vi "old - RT-R30.vi"() -> ()   [LabVIEW 2016]
uses:
  <vilib>/rvi/interface/nirviOpenFPGA/nirviOpenFPGA.xnode
  <vilib>/rvi/interface/nirviReadWriteControl/nirviReadWriteControl.xnode
  <vilib>/functionblocks/FB Property/FB Overlay DBL.ctl
  <vilib>/functionblocks/FB Core/FB Core.xnode
  <vilib>/functionblocks/Control/PID/PID.vi
  <vilib>/functionblocks/NI_FunctionBlock Libraries.lvlib
  FPGA-R30.vi
  <vilib>/Utility/error.llb/Error Cluster From Error Code.vi
  <vilib>/rvi/errors/niLvFpgaAdjustHostInterfaceError.vi
  NiFpgaLv.dll
  <vilib>/Instr/_visa.llb/VISA Configure Serial Port (Instr).vi
panel:
  in  "Ion gauge 3":T1
  in  "Tab Control":enum32{"Main", "Errors"}(tab)
  out "string":string
  out "Switch magnet field read":dbl
  out "switch magnet field":dbl(graph)
  out "Y Mag Steerer V":fxp<+/-,26,5> format="%.3g"
  out "Y magnet v":fxp<+/-,26,5> format="%.3g"
  out "X-I":fxp<+/-,26,5> format="%.3g"
  out "X- V":fxp<+/-,26,5> format="%.3g"
  out "X+ I":fxp<+/-,26,5> format="%.3g"
  out "X+ V":fxp<+/-,26,5> format="%.3g"
  out "R30 Quad B I":fxp<+/-,26,5> format="%.3g"
  out "R30 Quad A I":fxp<+/-,26,5> format="%.3g"
  out "ESA I":fxp<+/-,26,5> format="%.3g"
  out "ESA V":fxp<+/-,26,5> format="%.3g"
  out "Y-I":fxp<+/-,26,5> format="%.3g"
  out "Y-V":fxp<+/-,26,5> format="%.3g"
  out "Y+I":fxp<+/-,26,5> format="%.3g"
  out "Y+ V":fxp<+/-,26,5> format="%.3g"
  out "R30 Y Steerer":dbl
  out "HE Y+ (1)":dbl
  out "HE Y- (1)":dbl
  out "HE X+ (1)":dbl
  out "HE X- (1)":dbl
  out "HE Quad B":dbl
  out "HE Quad A":dbl
  out "ESA":dbl
  out "Analog input":fxp<+/-,26,5>[](array[numeric]) format="%.23g"
  out "analog output":fxp<+/-,64,32>[](array[numeric]) format="%.42g"
  out "Switch magnet AP 2":bool
  out "Switch magnet FC 2":bool
  out "Detector AP 2":bool
  out "Detector FC 2":bool
  out "Switch magnet FC IN 2":bool
  out "Switch magnet FC OUT 2":bool
  out "Detector FC OUT 2":bool
  out "Detector  FC IN 2":bool
  out "Det Ap IN 2":bool
  out "Det Ap OUT 2":bool
  out "Switch Ap OUT2 2":bool
  out "Switch Ap IN 2":bool
  out "match + rest of string":string
  out "x*y":dbl
  in  "derivative time (Td, min)":dbl=0.01
  in  "integral time (Ti, min)":dbl=0.01
  in  "proportional gain (Kc)":dbl=10.0
  out "Switch magnet field set":dbl
  out "Switch object tesla meter 2":u8[](array[numeric])
  out "Switch object tesla meter":u8[](array[numeric])
  out "R30 Detector Ion gauge 1":dbl
  out "R30 Detector Convectron gauge 1":dbl
  out "R30 ESA Ion gauge 1":dbl
  out "R30 ESA Convectron gauge 1":dbl
  out "Switch Image Ion Gauge 1":string
  out "Switch Image Convectron Gauge 1":string
  out "R30 ESA Convectron 1":string
  out "R30 ESA Ion Gauge 1":string
  out "R30 Detector Ion Gauge 1":string
  out "R30 Detector Convectron 1":string
  out "Y Mag Steerer I":fxp<+/-,26,5>
  out "Readback NSV loop error":errorcluster
  out "Sensor NSV error":errorcluster
  out "Actuator-Sensor Error":errorcluster
  out "Switch Mag Error 4":errorcluster
  out "Switch Mag Error 1":errorcluster
  out "Switch Mag Error 3":errorcluster
  out "Switch Mag Error 2":errorcluster
  out "Serial Connect Error":errorcluster
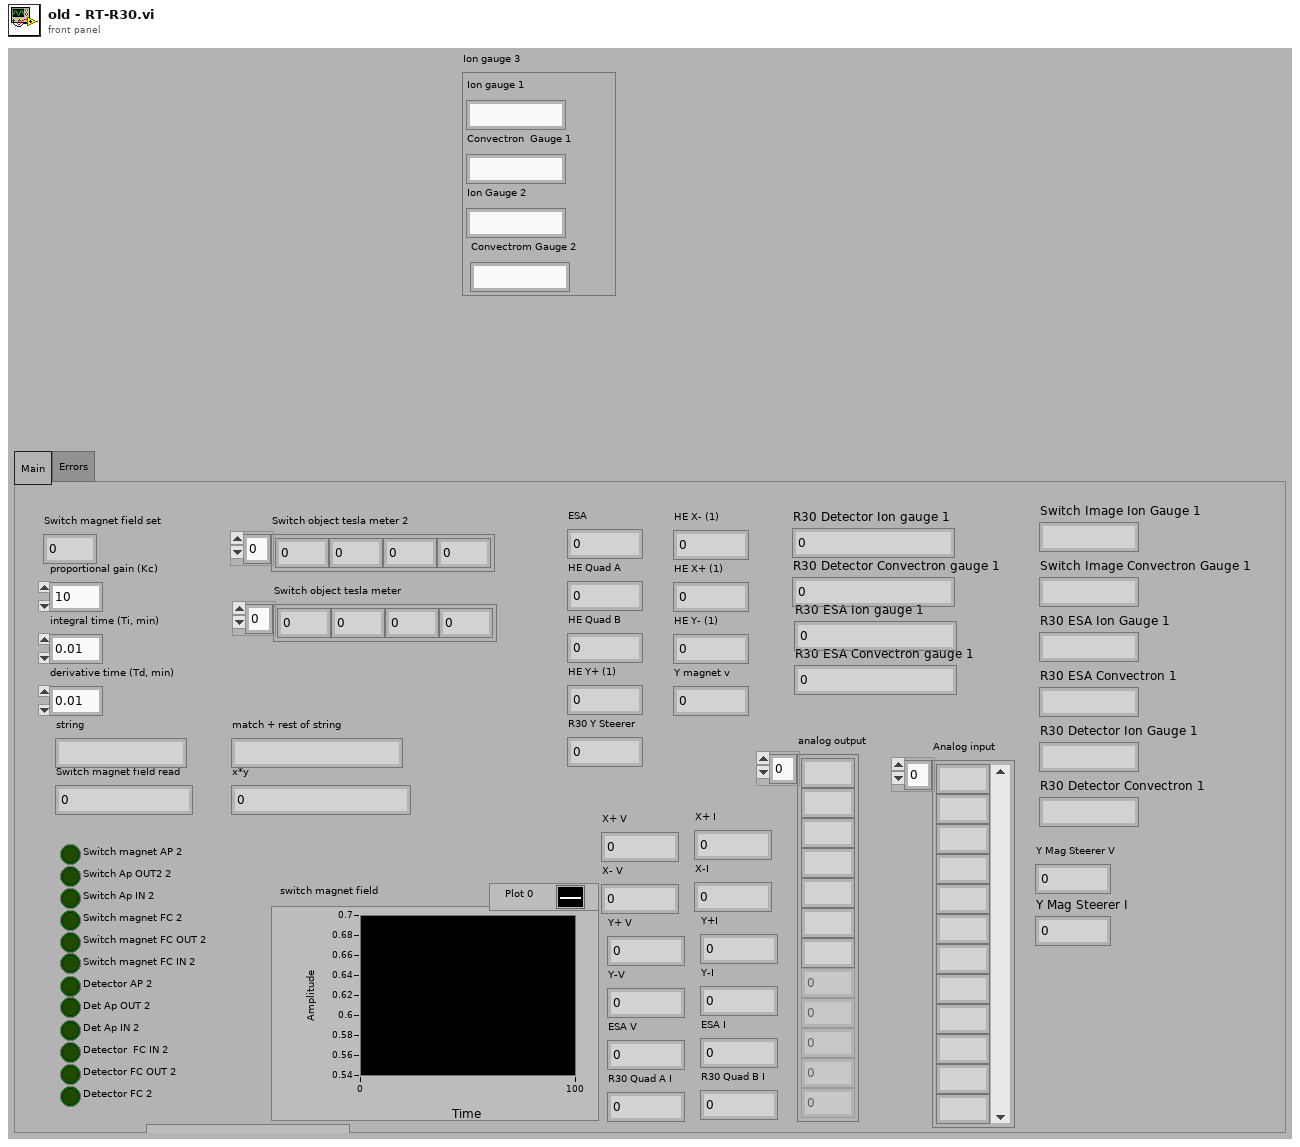
[diagram p1: front panel]
types:
  T1 = cluster{"Ion gauge 1":string, "Convectron  Gauge 1 ":string, "Ion Gauge 2":string, "Convectrom Gauge 2":string}
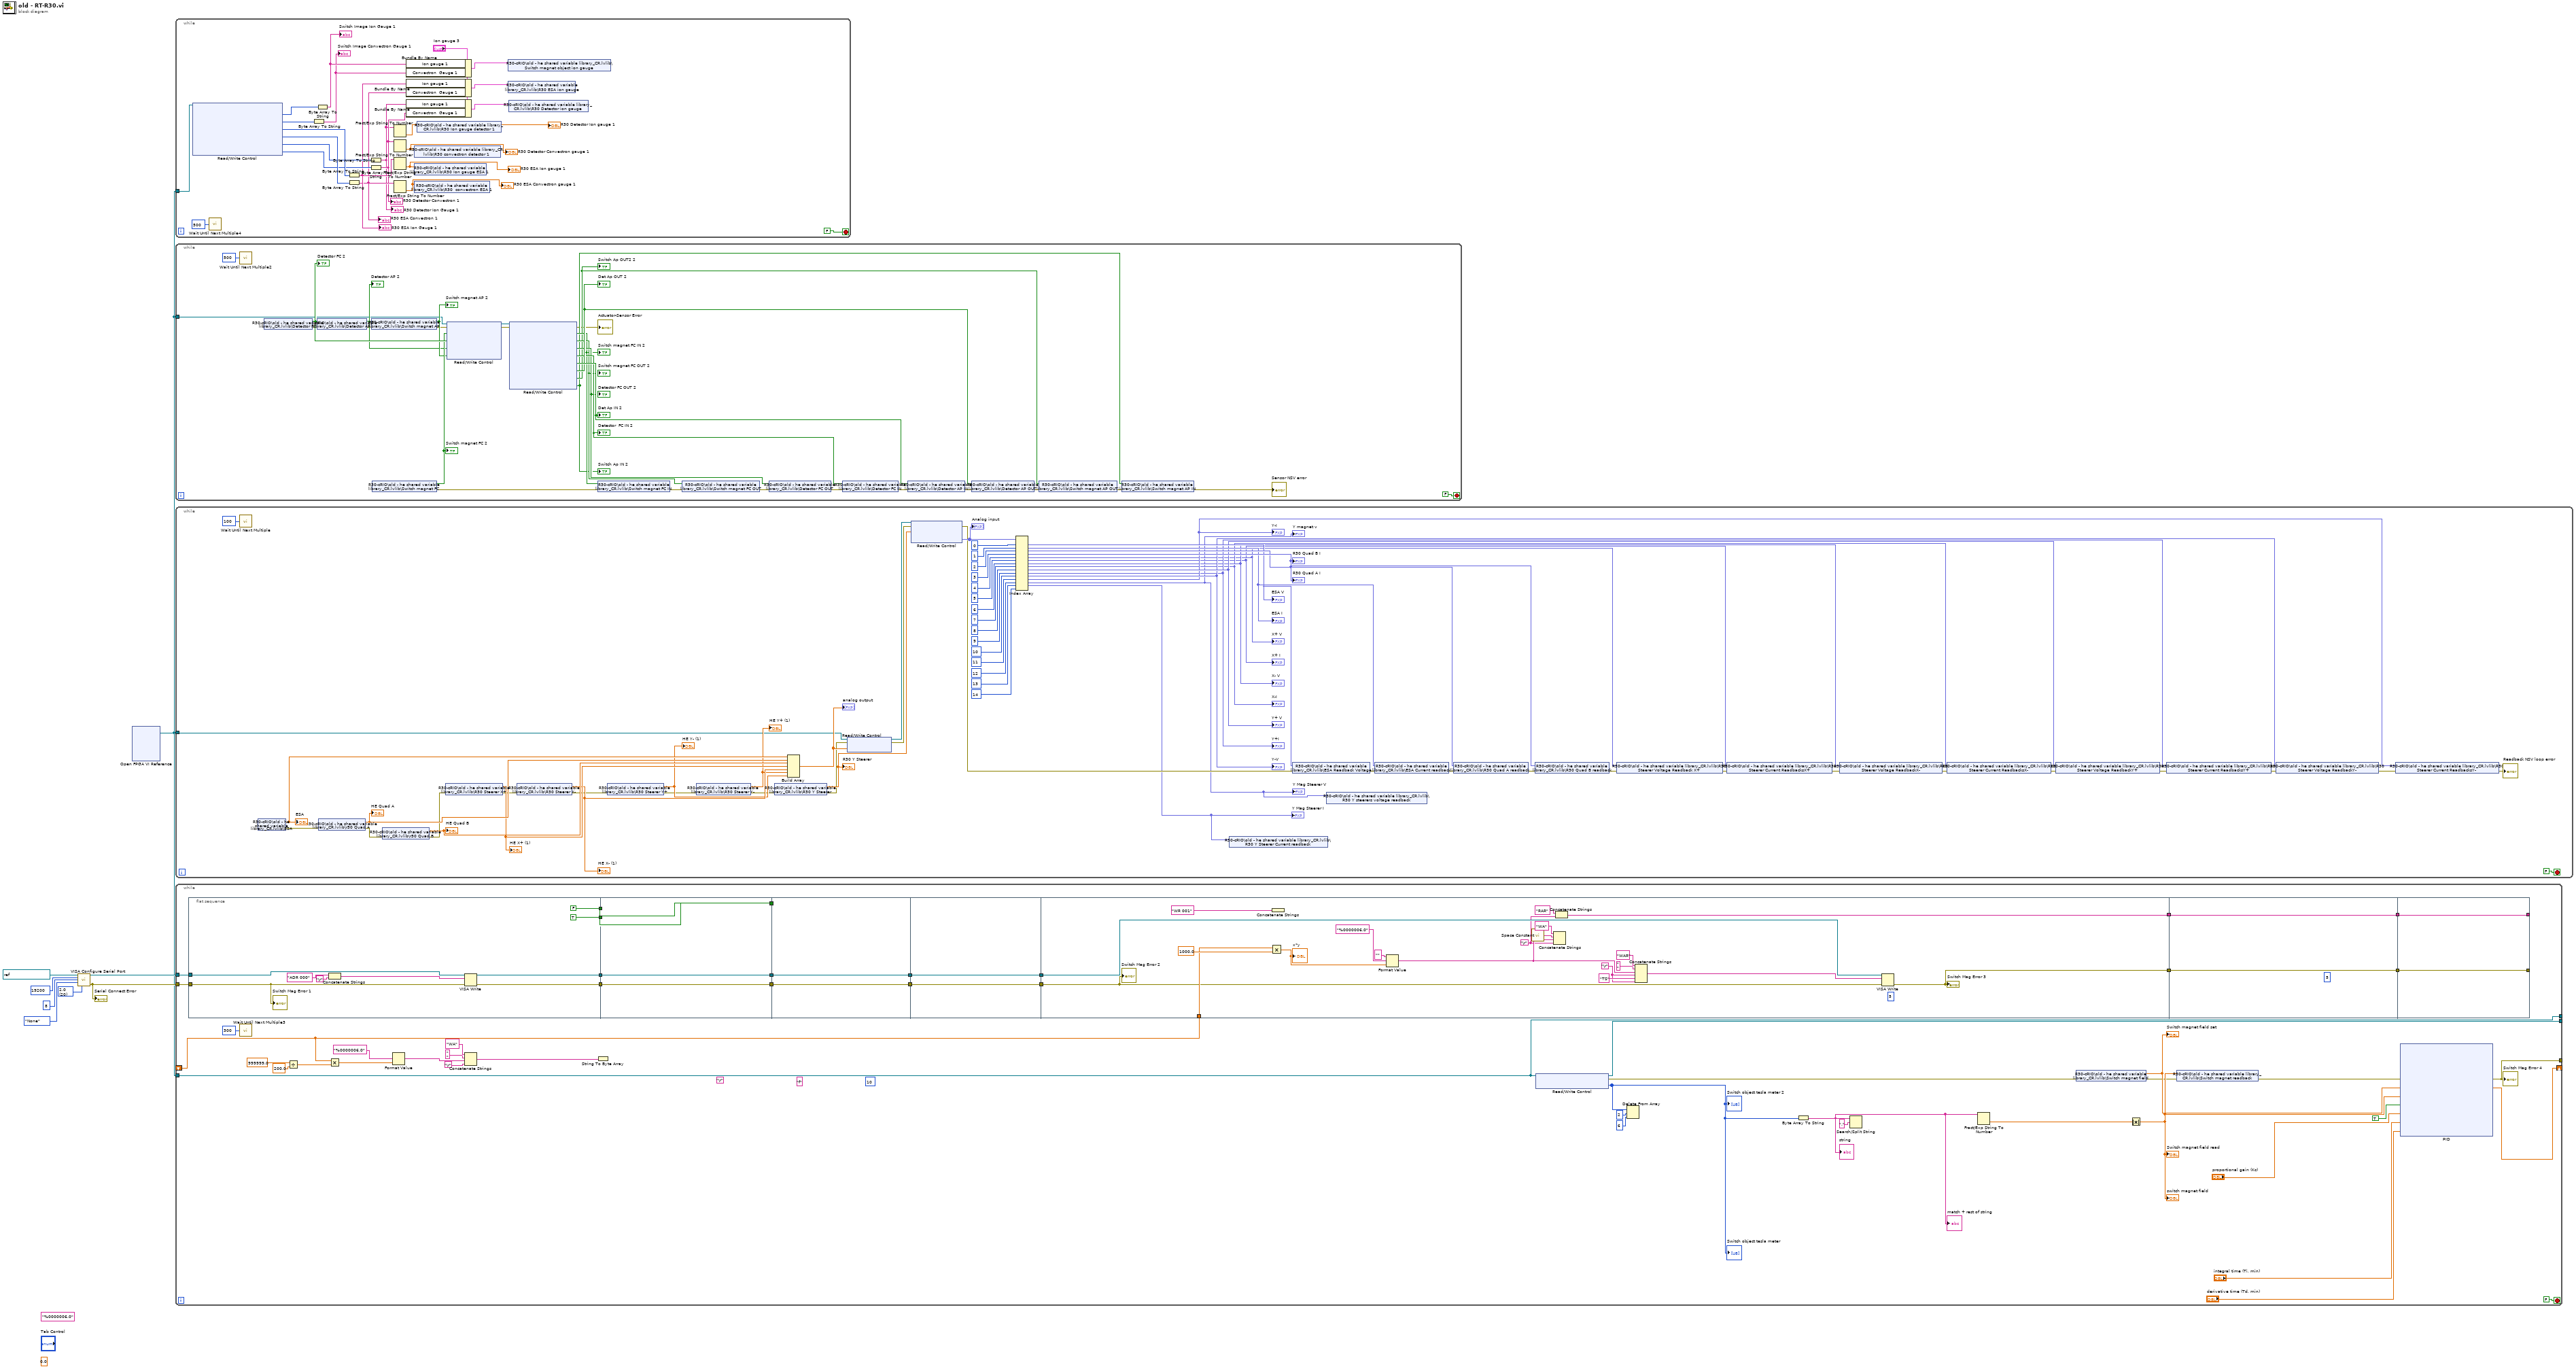
[diagram p0: block diagram]
diagram:
  w4 = u16 20 items=["1.0"=10, "1.5"=15, "2.0"=20] ("stop bits (10: 1 bit)")
  (unwired) 0.0 ("output")
  (unwired) "%0000006.0" ("format string")
  n1 = call-poly "VISA Configure Serial Port"("VISA resource name"=refnum<visa-resource-name> "ASRL1::INSTR", "baud rate (9600)"=u32 19200, "data bits (8)"=u16 8, "parity (0:none)"=enum16{"None", "Odd", "Even", "Mark", "Space"}."None", "stop bits (10: 1 bit)"=w4) -> ("VISA resource name out"=w3:refnum<visa-resource-name>, "error out"=w2:errorcluster)  [unwired: 9 in]
  "Serial Connect Error" <- w2
  n2 = xnode "Open FPGA VI Reference"() -> ("FPGA VI Reference Out"=w1:refnum<k20>)  [unwired: 2 in, 1 out]
  n3 = while {
    tunnel: w1 -> [w31]
    stop <- FALSE stop-if-true
    n4 = xnode "Read/Write Control"("FPGA VI Reference In"=w31) -> ("R30 Switch Image Ion gauge 1"=w19:u8[], "R30 Switch Image Convectron 1"=w20:u8[], "R30 ESA Ion gauge 1"=w24:u8[], "R30 ESA Convectron  1"=w23:u8[], "R30 Detector Ion gauge 1"=w22:u8[], "R30 Detector Convectron  1"=w21:u8[])  [unwired: 1 in, 2 out]
    n5 = call "Wait Until Next Multiple4"("Count(mSec)"=u32 500 ("Count(uSec)")) -> ()  [unwired: 1 out]
    n6 = Byte Array To String(unsigned byte array=w20) -> (string=w16:string)
    "Switch Image Convectron Gauge 1" <- w16
    n7 = Byte Array To String(unsigned byte array=w19) -> (string=w17:string)
    "Switch Image Ion Gauge 1" <- w17
    n8 = Byte Array To String(unsigned byte array=w24) -> (string=w15:string)
    "R30 ESA Ion Gauge 1" <- w15
    n9 = Byte Array To String(unsigned byte array=w23) -> (string=w14:string)
    "R30 ESA Convectron 1" <- w14
    n10 = Byte Array To String(unsigned byte array=w22) -> (string=w9:string)
    "R30 Detector Ion Gauge 1" <- w9
    n11 = Byte Array To String(unsigned byte array=w21) -> (string=w10:string)
    "R30 Detector Convectron 1" <- w10
    n12 = Fract/Exp String To Number(string=w9) -> (number=w28:dbl)  [unwired: 3 in, 1 out]
    "R30 Detector Ion gauge 1" <- w28
    n13 = Fract/Exp String To Number(string=w10) -> (number=w26:dbl)  [unwired: 3 in, 1 out]
    "R30 Detector Convectron gauge 1" <- w26
    n14 = Fract/Exp String To Number(string=w15) -> (number=w27:dbl)  [unwired: 3 in, 1 out]
    "R30 ESA Ion gauge 1" <- w27
    n15 = Fract/Exp String To Number(string=w14) -> (number=w25:dbl)  [unwired: 3 in, 1 out]
    "R30 ESA Convectron gauge 1" <- w25
    n16 = Bundle By Name(cluster="Ion gauge 3", "Ion gauge 1"=w17, "Convectron  Gauge 1"=w16) -> (w13:T1)
    n17 = Bundle By Name(cluster="Ion gauge 3", "Ion gauge 1"=w15, "Convectron  Gauge 1"=w14) -> (w12:T1)
    n18 = Bundle By Name(cluster="Ion gauge 3", "Ion gauge 1"=w9, "Convectron  Gauge 1"=w10) -> (w11:T1)
    n19 = shared-variable "R30-cRIO\\old - he shared variable library_CR.lvlib\\R30 convectron detector 1"(w26) -> ()  [unwired: 1 in, 1 out]
    n20 = shared-variable "R30-cRIO\\old - he shared variable library_CR.lvlib\\R30 Ion gauge ESA 1"(w27) -> ()  [unwired: 1 in, 1 out]
    n21 = shared-variable "R30-cRIO\\old - he shared variable library_CR.lvlib\\R30  convectron ESA 1"(w25) -> ()  [unwired: 1 in, 1 out]
    n22 = shared-variable "R30-cRIO\\old - he shared variable library_CR.lvlib\\R30 Ion gauge detector 1"(w28) -> ()  [unwired: 1 in, 1 out]
    n23 = shared-variable "R30-cRIO\\old - he shared variable library_CR.lvlib\\Switch magnet object ion gauge"(w13) -> ()  [unwired: 1 in, 1 out]
    n24 = shared-variable "R30-cRIO\\old - he shared variable library_CR.lvlib\\R30 ESA ion gauge"(w12) -> ()  [unwired: 1 in, 1 out]
    n25 = shared-variable "R30-cRIO\\old - he shared variable library_CR.lvlib\\R30 Detector ion gauge"(w11) -> ()  [unwired: 1 in, 1 out]
  }
  n26 = while {
    tunnel: w1 -> [w32]
    stop <- FALSE stop-if-true
    n27 = call "Wait Until Next Multiple2"("Count(mSec)"=u32 500 ("Count(uSec)")) -> ()  [unwired: 1 out]
    n28 = shared-variable "R30-cRIO\\old - he shared variable library_CR.lvlib\\Detector FC"() -> (w58:bool, error out=w36:errorcluster)  [unwired: 1 in]
    "Detector FC 2" <- w58
    n29 = shared-variable "R30-cRIO\\old - he shared variable library_CR.lvlib\\Detector AP"(error in=w36) -> (w55:bool, error out=w35:errorcluster)
    "Detector AP 2" <- w55
    n30 = shared-variable "R30-cRIO\\old - he shared variable library_CR.lvlib\\Switch magnet AP"(error in=w35) -> (w56:bool, error out=w34:errorcluster)
    "Switch magnet AP 2" <- w56
    n31 = shared-variable "R30-cRIO\\old - he shared variable library_CR.lvlib\\Switch magnet FC"() -> (w57:bool, error out=w44:errorcluster)  [unwired: 1 in]
    "Switch magnet FC 2" <- w57
    n32 = xnode "Read/Write Control"("FPGA VI Reference In"=w32, "error in"=w34, "Switch magnet FC"=w57, "Detector FC"=w58, "Detector AP"=w55, "Switch magnet ap"=w56) -> ("FPGA VI Reference Out"=w60:refnum<k20>, "error out"=w46:errorcluster)
    n33 = xnode "Read/Write Control"("FPGA VI Reference In"=w60, "error in"=w46) -> ("error out"=→"Actuator-Sensor Error":errorcluster, "Switch magnet FC IN"=w49:bool, "Switch magnet FC OUT"=w50:bool, "Detector FC OUT"=w51:bool, "Detector  FC IN"=w52:bool, "Det Ap IN"=w54:bool, "Det Ap OUT"=w53:bool, "Switch Ap OUT2"=w48:bool, "Switch Ap IN"=w47:bool)  [unwired: 1 out]
    "Switch magnet FC IN 2" <- w49
    "Switch magnet FC OUT 2" <- w50
    "Detector FC OUT 2" <- w51
    "Detector  FC IN 2" <- w52
    "Det Ap IN 2" <- w54
    "Det Ap OUT 2" <- w53
    "Switch Ap OUT2 2" <- w48
    "Switch Ap IN 2" <- w47
    n34 = shared-variable "R30-cRIO\\old - he shared variable library_CR.lvlib\\Switch magnet FC IN"(w49, error in=w44) -> (error out=w43:errorcluster)
    n35 = shared-variable "R30-cRIO\\old - he shared variable library_CR.lvlib\\Switch magnet FC OUT"(w50, error in=w43) -> (error out=w42:errorcluster)
    n36 = shared-variable "R30-cRIO\\old - he shared variable library_CR.lvlib\\Detector FC OUT"(w51, error in=w42) -> (error out=w41:errorcluster)
    n37 = shared-variable "R30-cRIO\\old - he shared variable library_CR.lvlib\\Detector FC IN"(w52, error in=w41) -> (error out=w40:errorcluster)
    n38 = shared-variable "R30-cRIO\\old - he shared variable library_CR.lvlib\\Detector AP IN"(w54, error in=w40) -> (error out=w39:errorcluster)
    n39 = shared-variable "R30-cRIO\\old - he shared variable library_CR.lvlib\\Detector AP OUT"(w53, error in=w39) -> (error out=w38:errorcluster)
    n40 = shared-variable "R30-cRIO\\old - he shared variable library_CR.lvlib\\Switch magnet AP OUT"(w48, error in=w38) -> (error out=w37:errorcluster)
    n41 = shared-variable "R30-cRIO\\old - he shared variable library_CR.lvlib\\Switch magnet AP IN"(w47, error in=w37) -> (error out=→"Sensor NSV error":errorcluster)
  }
  n42 = while {
    tunnel: w1 -> [w88]
    stop <- FALSE stop-if-true
    n43 = call "Wait Until Next Multiple"("Count(mSec)"=u32 100 ("Count(uSec)")) -> ()  [unwired: 1 out]
    n44 = shared-variable "R30-cRIO\\old - he shared variable library_CR.lvlib\\ESA"() -> (w125:dbl, error out=w85:errorcluster)  [unwired: 1 in]
    "ESA" <- w125
    n45 = shared-variable "R30-cRIO\\old - he shared variable library_CR.lvlib\\r30 Quad A"(error in=w85) -> (w124:dbl, error out=w84:errorcluster)
    "HE Quad A" <- w124
    n46 = shared-variable "R30-cRIO\\old - he shared variable library_CR.lvlib\\r30 Quad B"(error in=w84) -> (w123:dbl, error out=w83:errorcluster)
    "HE Quad B" <- w123
    n47 = shared-variable "R30-cRIO\\old - he shared variable library_CR.lvlib\\R30 Steerer X+"(error in=w83) -> (w122:dbl, error out=w82:errorcluster)
    "HE X+ (1)" <- w122
    n48 = shared-variable "R30-cRIO\\old - he shared variable library_CR.lvlib\\R30 Steerer X-"(error in=w82) -> (w121:dbl, error out=w81:errorcluster)
    "HE X- (1)" <- w121
    n49 = shared-variable "R30-cRIO\\old - he shared variable library_CR.lvlib\\R30 Steerer Y+"(error in=w81) -> (w120:dbl, error out=w80:errorcluster)
    "HE Y- (1)" <- w120
    n50 = shared-variable "R30-cRIO\\old - he shared variable library_CR.lvlib\\R30 Steerer Y-"(error in=w80) -> (w119:dbl, error out=w79:errorcluster)
    "HE Y+ (1)" <- w119
    n51 = shared-variable "R30-cRIO\\old - he shared variable library_CR.lvlib\\R30 Y Steerer"(error in=w79) -> (w91:dbl, error out=w78:errorcluster)
    "R30 Y Steerer" <- w91
    n52 = Build Array(w125, w124, w123, w122, w121, w119, w120) -> (w90:dbl[])
    "analog output" <- w90
    n53 = xnode "Read/Write Control"("FPGA VI Reference In"=w88, "error in"=w78, "analog output"=w90) -> ("FPGA VI Reference Out"=w118:refnum<k20>, "error out"=w86:errorcluster)
    n54 = xnode "Read/Write Control"("FPGA VI Reference In"=w118, "error in"=w86, "y steerer magnet"=w91) -> ("error out"=w77:errorcluster, "analog readback"=w87:fxp<+/-,26,5>[])  [unwired: 1 out]
    "Analog input" <- w87
    n55 = Index Array(array=w87, index #1=0 ("index"), index #2=1 ("index"), index #3=2 ("index"), index #4=3 ("index"), index #5=4 ("index"), index #6=5 ("index"), index #7=6 ("index"), index #8=7 ("index"), index #9=8 ("index"), index #10=9 ("index"), index #11=10 ("index"), index #12=11 ("index"), index #13=12 ("index"), index #14=13 ("index"), index #15=14 ("index")) -> (element #1=w102:fxp<+/-,26,5>, element #2=w103:fxp<+/-,26,5>, element #3=w104:fxp<+/-,26,5>, element #4=w105:fxp<+/-,26,5>, element #5=w95:fxp<+/-,26,5>, element #6=w94:fxp<+/-,26,5>, element #7=w97:fxp<+/-,26,5>, element #8=w96:fxp<+/-,26,5>, element #9=w101:fxp<+/-,26,5>, element #10=w98:fxp<+/-,26,5>, element #11=w100:fxp<+/-,26,5>, element #12=w99:fxp<+/-,26,5>, element #13=w63:fxp<+/-,26,5>, element #14=w62:fxp<+/-,26,5>)  [unwired: 1 out]
    "Y+ V" <- w101
    "Y+I" <- w98
    "Y-V" <- w100
    "Y-I" <- w99
    "ESA V" <- w102
    "ESA I" <- w103
    "R30 Quad A I" <- w104
    "R30 Quad B I" <- w105
    "X+ V" <- w95
    "X+ I" <- w94
    "X- V" <- w97
    "X-I" <- w96
    "Y magnet v" <- w63
    "Y Mag Steerer V" <- w63
    "Y Mag Steerer I" <- w62
    n56 = shared-variable "R30-cRIO\\old - he shared variable library_CR.lvlib\\R30 Y Steerer Current readback"(w62) -> ()  [unwired: 1 in, 1 out]
    n57 = shared-variable "R30-cRIO\\old - he shared variable library_CR.lvlib\\ESA Readback Voltage"(w102, error in=w77) -> (error out=w76:errorcluster)
    n58 = shared-variable "R30-cRIO\\old - he shared variable library_CR.lvlib\\R30 Y steerers voltage readback"(w63) -> ()  [unwired: 1 in, 1 out]
    n59 = shared-variable "R30-cRIO\\old - he shared variable library_CR.lvlib\\ESA Current readback"(w103, error in=w76) -> (error out=w75:errorcluster)
    n60 = shared-variable "R30-cRIO\\old - he shared variable library_CR.lvlib\\R30 Quad A readback"(w104, error in=w75) -> (error out=w74:errorcluster)
    n61 = shared-variable "R30-cRIO\\old - he shared variable library_CR.lvlib\\R30 Quad B readback"(w105, error in=w74) -> (error out=w73:errorcluster)
    n62 = shared-variable "R30-cRIO\\old - he shared variable library_CR.lvlib\\R30 Steerer Voltage Readback X+"(w95, error in=w73) -> (error out=w72:errorcluster)
    n63 = shared-variable "R30-cRIO\\old - he shared variable library_CR.lvlib\\R30 Steerer Current ReadbacksX+"(w94, error in=w72) -> (error out=w71:errorcluster)
    n64 = shared-variable "R30-cRIO\\old - he shared variable library_CR.lvlib\\R30 Steerer Voltage ReadbackX-"(w97, error in=w71) -> (error out=w70:errorcluster)
    n65 = shared-variable "R30-cRIO\\old - he shared variable library_CR.lvlib\\R30 Steerer Current ReadbacksX-"(w96, error in=w70) -> (error out=w69:errorcluster)
    n66 = shared-variable "R30-cRIO\\old - he shared variable library_CR.lvlib\\R30 Steerer Voltage ReadbackY+"(w101, error in=w69) -> (error out=w68:errorcluster)
    n67 = shared-variable "R30-cRIO\\old - he shared variable library_CR.lvlib\\R30 Steerer Current ReadbacksY+"(w98, error in=w68) -> (error out=w67:errorcluster)
    n68 = shared-variable "R30-cRIO\\old - he shared variable library_CR.lvlib\\R30 Steerer Voltage ReadbackY-"(w100, error in=w67) -> (error out=w66:errorcluster)
    n69 = shared-variable "R30-cRIO\\old - he shared variable library_CR.lvlib\\R30 Steerer Current ReadbacksY-"(w99, error in=w66) -> (error out=→"Readback NSV loop error":errorcluster)
  }
  n70 = while {
    tunnel: [w132] -> _
    tunnel: [w138] -> _
    shift-right: [w170] -> _
    shift-left: _ -> [w139]
    tunnel: [w131] -> _
    tunnel: w2 -> [w142]
    tunnel: w3 -> [w141]
    tunnel: w1 -> [w131]
    stop <- FALSE stop-if-true
    (unwired) "\r"
    (unwired) u32 10 ("byte count")
    (unwired) "f" ("write buffer")
    n71 = flat-sequence {
      tunnel: [w181] -> w158
      tunnel: [TRUE ("Communications On/Off")] -> w157
      tunnel: [FALSE ("Communications Mode")] -> w156
      tunnel: [w179] -> w155
      tunnel: w142 -> [w177]
      tunnel: w141 -> [w178]
      tunnel: w158 -> [w189]
      tunnel: [w189] -> w154
      tunnel: [w188] -> w153
      tunnel: w157 -> [w188]
      tunnel: w156 -> [w187]
      tunnel: [w187] -> w152
      tunnel: [w186] -> w151
      tunnel: w155 -> [w186]
      tunnel: w154 -> [w190]
      tunnel: w153 -> [_]
      tunnel: w152 -> [_]
      tunnel: [w190] -> w150
      tunnel: w151 -> [w191]
      tunnel: [w191] -> w149
      tunnel: w150 -> [w193]
      tunnel: [w193] -> w148
      tunnel: [w192] -> w147
      tunnel: w149 -> [w192]
      tunnel: w148 -> [w206]
      tunnel: [w200] -> w146
      tunnel: w147 -> [w195]
      tunnel: [w201] -> w145
      tunnel: w139 -> [w202]
      tunnel: w146 -> [w215]
      tunnel: [w214] -> w144
      tunnel: w145 -> [w214]
      tunnel: [w215] -> w143
      tunnel: w144 -> [w216]
      tunnel: w143 -> [w217]
      tunnel: [w217] -> _
      tunnel: [w216] -> _
      frame #0 {
        n72 = Concatenate Strings("ADR 000" ("Write String"), "\r") -> (w180:string)
        n73 = VISA Write(VISA resource name=w178, write buffer=w180, error in (no error)=w177) -> (VISA resource name out=w181:refnum<visa-resource-name>, error out=w179:errorcluster)  [unwired: 1 out]
        "Switch Mag Error 1" <- w177
      }
      frame #1 {
      }
      frame #2 {
      }
      frame #3 {
      }
      frame #4 {
        (unwired) u32 5 ("byte count")
        w196 = "\r"
        w209 = "\r"
        n74 = Multiply(x=w202, y=1000.0) -> (x*y=w203:dbl)
        "x*y" <- w203
        n75 = Concatenate Strings("WR 001" ("Write String")) -> ()  [unwired: 1 out]
        n76 = Format Value(string ("")="", format string="%0000006.0", value (0)=w203) -> (output string=w197:string)
        n77 = call <vilib>:"Space Constant.vi"() -> ("String"=w198:string)
        n78 = Concatenate Strings("WA" ("Write String"), w198, w197, w196) -> ()  [unwired: 1 out]
        n79 = Concatenate Strings("RAR" ("Write String"), w196) -> (w200:string)
        n80 = Concatenate Strings("WAR", " ", w197, w209, "TS" ("string"), w209) -> (w194:string)
        n81 = VISA Write(VISA resource name=w206, write buffer=w194, error in (no error)=w195) -> (error out=w201:errorcluster)  [unwired: 2 out]
        "Switch Mag Error 3" <- w201
        "Switch Mag Error 2" <- w195
      }
      frame #5 {
        (unwired) u32 5 ("byte count")
      }
      frame #6 {
      }
    }
    n82 = call "Wait Until Next Multiple3"("Count(mSec)"=u32 300 ("millisecond multiple")) -> ()  [unwired: 1 out]
    n83 = Divide(x=999999.0, y=200.0) -> (x/y=w174:dbl)
    n84 = Multiply(x=w139, y=w174) -> (x*y=w140:dbl)
    n85 = Format Value(format string="%0000006.0", value (0)=w140) -> (output string=w159:string)  [unwired: 1 out]
    n86 = Concatenate Strings("WA", " ", w159, "\r") -> (w161:string)
    n87 = String To Byte Array(string=w161) -> ()  [unwired: 1 out]
    n88 = xnode "Read/Write Control"("FPGA VI Reference In"=w131) -> ("FPGA VI Reference Out"=w138:refnum<k20>, "error out"=w135:errorcluster, "Switch object tesla meter"=w130:u8[])  [unwired: 1 in]
    "Switch object tesla meter" <- w130
    "Switch object tesla meter 2" <- w130
    n89 = Delete From Array(array=w130, length=2, index=6) -> ()  [unwired: 2 out]
    n90 = Byte Array To String(unsigned byte array=w130) -> (string=w127:string)
    "string" <- w127
    "match + rest of string" <- w127
    n91 = Search/Split String(string=w127, search string/char (-)=".") -> ()  [unwired: 4 out]
    n92 = Fract/Exp String To Number(string=w127) -> (number=w136:dbl)  [unwired: 3 in, 1 out]
    n93 = shared-variable "R30-cRIO\\old - he shared variable library_CR.lvlib\\Switch magnet field"(error in=w135) -> (w168:dbl, error out=w134:errorcluster)
    "Switch magnet field set" <- w168
    n94 = Absolute Value(x=w136) -> (abs(x)=w137:dbl)
    "Switch magnet field read" <- w137
    "switch magnet field" <- w137
    n95 = shared-variable "R30-cRIO\\old - he shared variable library_CR.lvlib\\Switch magnet readback"(w137, error in=w134) -> (error out=w133:errorcluster)
    n96 = xnode "PID"("error in"=w133, "setpoint"=w168, "process variable"=w137, "auto? (T)"=TRUE, "proportional gain (Kc)"="proportional gain (Kc)", "integral time (Ti, min)"="integral time (Ti, min)", "derivative time (Td, min)"="derivative time (Td, min)") -> ("error out"=w132:errorcluster, "output"=w170:dbl)
    "Switch Mag Error 4" <- w132
  }
